vi "MGI Get Executable Version.vi"() -> (2 "Version":string)   [LabVIEW 2016]
doc: "If this VI is built into an executable, it returns the file version (this is the number typed into the application builder for LabVIEW built exes. When run in the development environment it simply returns \"Development\". Executables created with versions of LabVIEW earlier than 8.0 do not include the necessary information in the executable for this VI to return the version.\n\nAuthored by Robert C. Mortensen\nsupport@mooregoodideas.com\nwww.mooregoodideas.com\n\nCopyright (c) 2010, Moore Good Ideas, Inc.\n\nAll rights reserved.\n\nRedistribution and use in source and binary forms, with or without modification, are permitted provided that the following conditions are met:\n\n * Redistributions of source code must retain the above copyright notice, this list of conditions and the following disclaimer.\n * Redistributions in binary form must reproduce the above copyright notice, this list of conditions and the following disclaimer in the documentation and/or other materials provided with the distribution.\n * Neither the name of Moore Good Ideas, Inc. nor the names of its contributors may be used to endorse or promote products derived from this software without specific prior written permission.\n\nTHIS SOFTWARE IS PROVIDED BY THE COPYRIGHT HOLDERS AND CONTRIBUTORS \"AS IS\" AND ANY EXPRESS OR IMPLIED WARRANTIES, INCLUDING, BUT NOT LIMITED TO, THE IMPLIED WARRANTIES OF MERCHANTABILITY AND FITNESS FOR A PARTICULAR PURPOSE ARE DISCLAIMED. IN NO EVENT SHALL THE COPYRIGHT OWNER OR CONTRIBUTORS BE LIABLE FOR ANY DIRECT, INDIRECT, INCIDENTAL, SPECIAL, EXEMPLARY, OR CONSEQUENTIAL DAMAGES (INCLUDING, BUT NOT LIMITED TO, PROCUREMENT OF SUBSTITUTE GOODS OR SERVICES; LOSS OF USE, DATA, OR PROFITS; OR BUSINESS INTERRUPTION) HOWEVER CAUSED AND ON ANY THEORY OF LIABILITY, WHETHER IN CONTRACT, STRICT LIABILITY, OR TORT (INCLUDING NEGLIGENCE OR OTHERWISE) ARISING IN ANY WAY OUT OF THE USE OF THIS SOFTWARE, EVEN IF ADVISED OF THE POSSIBILITY OF SUCH DAMAGE."
uses:
  version.dll
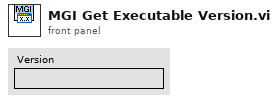
[diagram p1: front panel]
types:
  T1 = enum32{"invalid app kind", "Development System", "Run Time System", "Student Edition", "Embedded LabVIEW", "Evaluation", "Custom"}
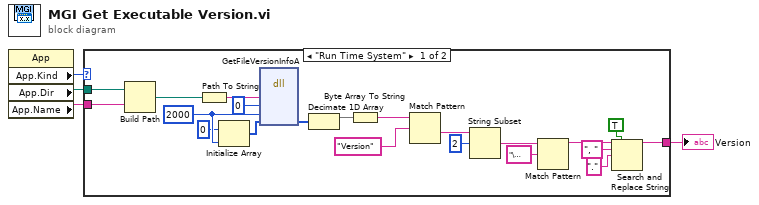
[diagram p0: block diagram]
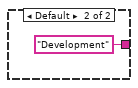
[diagram p2: hidden frame]
diagram:
  n1 = property class="App"() -> ("App.Kind"=w2:T1, "App.Dir"=w3:path, "App.Name"=w4:string)  [unwired: 2 in, 2 out]
  n2 = case shown="\"Run Time System\"" w2 {
    tunnel: w4 -> [w25 _]
    tunnel: w3 -> [w24 _]
    tunnel: [w5 "Development" ("pattern label")] -> w1
    frame "Run Time System" {
      w13 = u32 2000 ("dwLen")
      n3 = Build Path(base path=w24, name or relative path=w25) -> (appended path=w6:path)
      n4 = Path To String(path=w6) -> (string=w8:string)
      n5 = Initialize Array(u8 0 ("element"), w13) -> (w10:u8[])
      n6 = dll-call lib="version.dll" fn="GetFileVersionInfoA"("lptstrFilename"=w8, "dwHandle"=0, "dwLen"=w13, "lpData"=w10) -> ("lpData"=w11:u8[])  [unwired: 7 in, 2 out]
      n7 = Decimate 1D Array(w11) -> (w12:u8[])  [unwired: 1 out]
      n8 = Byte Array To String(unsigned byte array=w12) -> (string=w14:string)
      n9 = Match Pattern(string=w14, regular expression="Version") -> (after substring=w16:string)  [unwired: 1 in, 3 out]
      n10 = String Subset(string=w16, offset (0)=2) -> (substring=w18:string)  [unwired: 1 in]
      n11 = Match Pattern(string=w18, regular expression="\u0000") -> (before substring=w20:string)  [unwired: 1 in, 3 out]
      n12 = Search and Replace String(replace all?=TRUE ("replace all? (F)"), input string=w20, search string=", ", replace string="." ("replace string (\"\")")) -> (result string=w5:string)  [unwired: 4 in, 3 out]
    }
    frame Default {
    }
  }
  "Version" <- w1
